vi "HW_Gantner_DAQ FGV.vi"(0 "DevName":string="Gantner", 1 "Oper.":T13, 2 "Path.ModuCFG":path, 5 "ActiveModuTag":string, 7 "TreePara":cluster{"ColHdrs":string[], "Items":string[][]}, 9 "DataBuf":refnum<queue>, 11 "error in":errorcluster caption="错误输入", 12 "ImportPara":T1(array[cluster])) -> (3 "Cfg out":T3[](array[typedef]), 4 "ActiveModuCHtype":string, 6 "Modu[] info":T2[](array[typedef]), 8 "ActiveCFG":T3, 10 "cfg change?":bool, 14 "TempCFG out":T3[](array[typedef]), 15 "error out":errorcluster caption="错误输出")   [LabVIEW 2016]
uses:
  DAQ FGV Operations.ctl
  Ctrls/HardWare _ Module Configuration.ctl
  Ctrls/HardWare _ Channel Parameters.ctl
  GantnerDriver/Gantner-Instruments HighSpeedPort/e.gate Configuration.ctl
  GantnerDriver/Gantner-Instruments HighSpeedPort/e.gate Channel Data.ctl
  GantnerDriver/Gantner-Instruments HighSpeedPort/e.gate Data Type.ctl
  GantnerDriver/Gantner-Instruments HighSpeedPort/e.gate Protocol Type.ctl
  GantnerDriver/Gantner-Instruments HighSpeedPort/e.gate Module  Data.ctl
  GantnerDriver/Gantner-Instruments HighSpeedPort/e.gateHSP_DLLhandle.ctl
  Gantner Device Info.ctl
  HW_Module Info.ctl
  Ctrls/HardWare Basic Info _ Channel.ctl
  X-DAQ Viewer/Controls/ConfigFGVCtrl.ctl
panel:
  in  "tempVari":T11={"DevName"="", "Usedcfg"=[], "TempCFG"=[], "ActiveModuIdx"=0, "SampRate"=0.0, "T0"=timestamp(0 s since 1904-01-01), "Path"={"ModuCFG_dflt"=path "", "ModuCFG_InUsed"=path ""}, "AllInUsedModu[]"=[], "Configuration"={"connection ID"=refnum, "IPAddress"="", "BufferIndex"=0, "StateMessage"="", "StateCode"=0, "HeaderSize"=0, "BufferSize"=0, "IsBigEndian"=0, "Version"=0, "ChannelCount"=0, "FrameLength"=0, "StartTime"=0.0, "dActTimeToSecondFactor"=0.0, "StartTimeToDayFactor"=0.0, "BufferFillRate"=0.0, "SampleRate"=0.0, "ChannelData"=[], "DecodeTimeFormat"="", "SummaryPath"="", "WithCheckSum"=0, "dActTimeDataType"=enum."NO", "MaxWriteCount"=0, "MaxReadCount"=0, "TempOffsetRead"=0, "TempLengthRead"=0, "Protocol"=enum."ASCII", "IsSupported"=0, "InputAccessList"=[], "OutputAccessList"=[], "DataSource"=enum."CircleBuffer", "Modules"=[], "DLL-Handle"={"clientInstance"=0, "connectionInstance"=0}}, "Iteration"=1000, "InUsedPhyCH[]"={"CHAlias"=[], "Unit"=[], "SampleRate"=[], "FilterFreq"=[], "SlopeA"=[], "InterceptB"=[], "SampMax"=[], "SampMin"=[], "AlarmMax"=[], "AlarmMin"=[], "Formula"=[]}, "StartT0"=timestamp(0 s since 1904-01-01), "Modu[] info"=[], "InUsedChanIdx[]"=[], "Wait (ms)"=500, "PhyChUsed[]"=[]} {"Configuration"."StartTime" format="%#.10f"; "Configuration"."dActTimeToSecondFactor" format="%#.10f"; "Configuration"."StartTimeToDayFactor" format="%#_10f"}
  in  "CFGinTree":T12
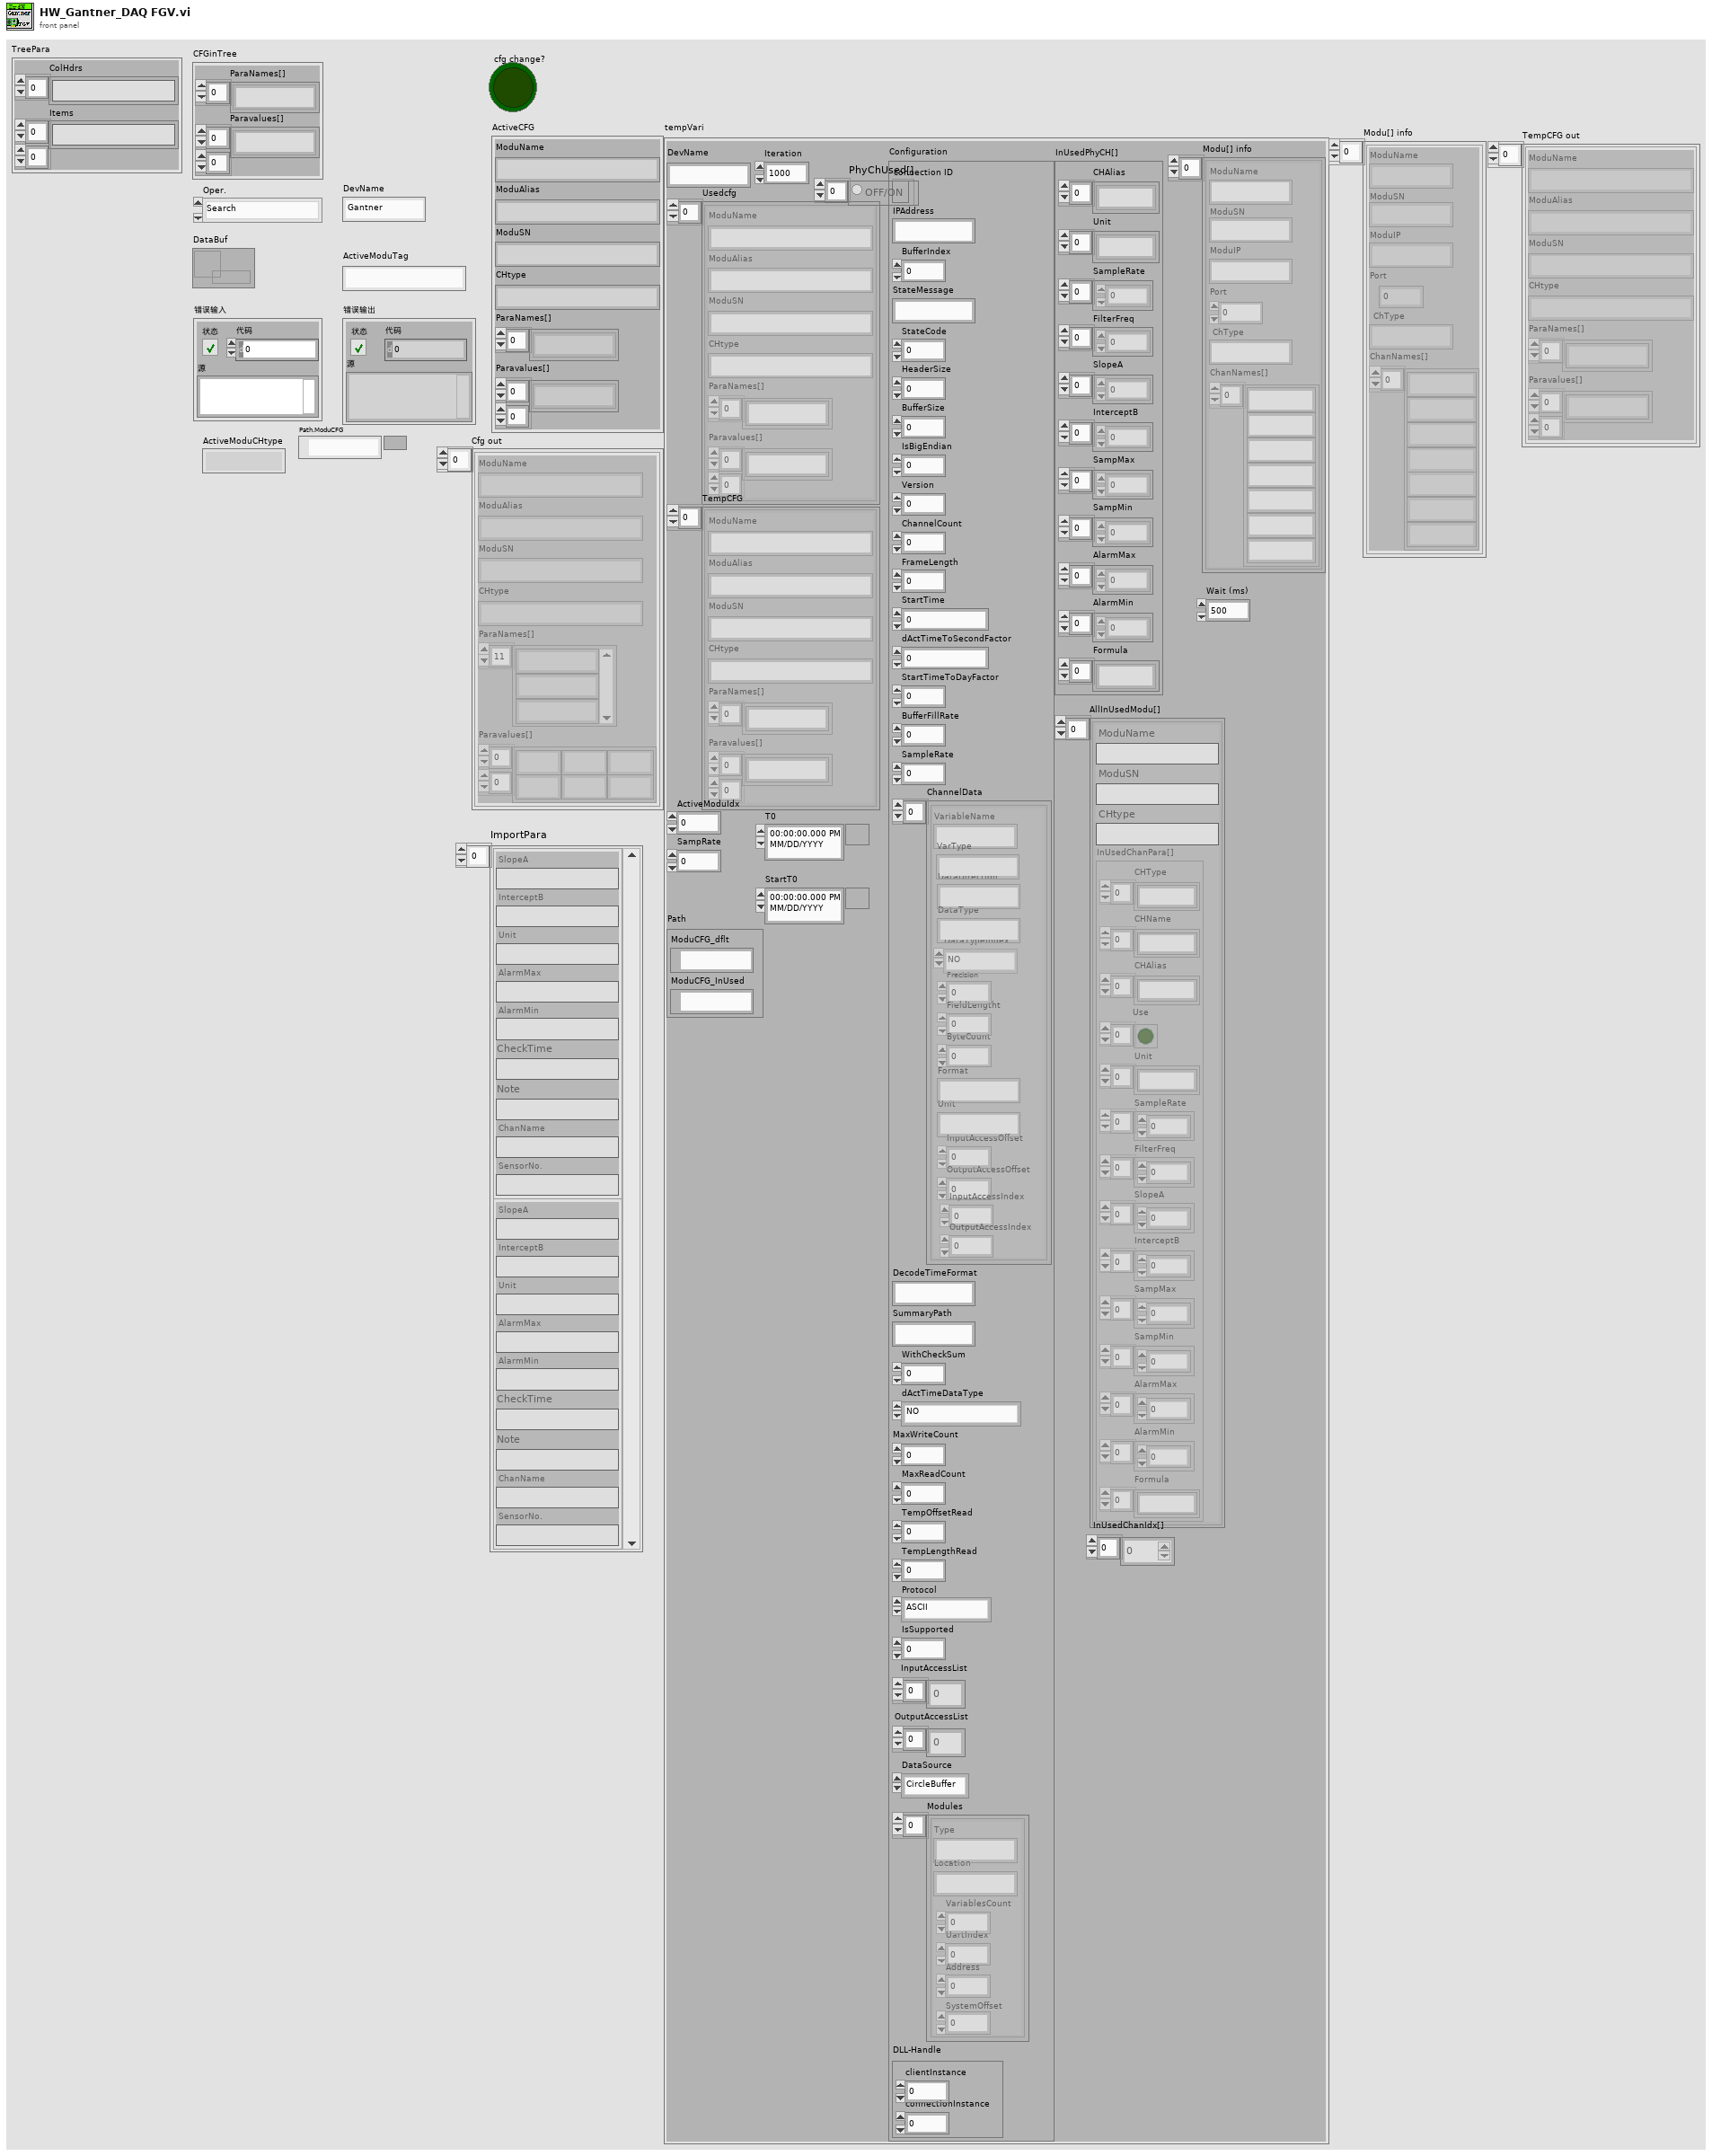
[diagram p1: front panel]
types:
  T1 = cluster{"SlopeA":string, "InterceptB":string, "Unit":string, "AlarmMax":string, "AlarmMin":string, "CheckTime":string, "Note":string, "ChanName":string, "SensorNo.":string}[]
  T2 = typedef "Gantner Device Info.ctl" = cluster{"ModuName":string, "ModuSN":string, "ModuIP":string, "Port":i32, "ChType":string, "ChanNames[]":string[]}
  T3 = typedef "HardWare _ Module Configuration.ctl" = cluster{"ModuName":string, "ModuAlias":string, "ModuSN":string, "CHtype":string, "ParaNames[]":string[], "Paravalues[]":string[][]}
  T4 = typedef "HardWare _ Channel Parameters.ctl" = cluster{"CHType":string[], "CHName":string[], "CHAlias":string[], "Use":bool[], "Unit":string[], "SampleRate":dbl[], "FilterFreq":dbl[], "SlopeA":dbl[], "InterceptB":dbl[], "SampMax":dbl[], "SampMin":dbl[], "AlarmMax":dbl[], "AlarmMin":dbl[], "Formula":string[]}
  T5 = typedef "e.gate Configuration.ctl" = cluster{"connection ID":refnum<k5>, "IPAddress":string, "BufferIndex":i32, "StateMessage":string, "StateCode":i8, "HeaderSize":i32, "BufferSize":i32, "IsBigEndian":i32, "Version":i32, "ChannelCount":i32, "FrameLength":i32, "StartTime":dbl, "dActTimeToSecondFactor":dbl, "StartTimeToDayFactor":dbl, "BufferFillRate":dbl, "SampleRate":dbl, "ChannelData":T6[], "DecodeTimeFormat":string, "SummaryPath":string, "WithCheckSum":i32, "dActTimeDataType":T7, "MaxWriteCount":i32, "MaxReadCount":i32, "TempOffsetRead":i32, "TempLengthRead":i32, "Protocol":T8, "IsSupported":i32, "InputAccessList":i32[], "OutputAccessList":i32[], "DataSource":enum16{"CircleBuffer", "test.con Logger", "test.con Archive"}, "Modules":T9[], "DLL-Handle":T10}
  T6 = typedef "e.gate Channel Data.ctl" = cluster{"VariableName":string, "DataDirection":string, "DataType":string, "DataTypeIndex":T7, "Precision":i16, "FieldLengtht":i16, "ByteCount":i32, "Format":string, "Unit":string, "InputAccessOffset":i32, "OutputAccessOffset":i16, "InputAccessIndex":i16, "OutputAccessIndex":i16, "VarType":string}
  T7 = typedef "e.gate Data Type.ctl" = enum16{"NO", "BOOL", "SINT8", "USINT8", "SINT16", "USINT16", "SINT32", "USINT32", "FLOAT", "SET8", "SET16", "SET32", "DOUBLE", "SINT64", "USINT64", "SET64"}
  T8 = typedef "e.gate Protocol Type.ctl" = enum16{"ASCII", "HighspeedPort Online", "HighspeedPort Buffer", "eGateHighspeedPortDLL "}
  T9 = typedef "e.gate Module  Data.ctl" = cluster{"Type":string, "Location":string, "VariablesCount":i16, "UartIndex":i16, "Address":i16, "SystemOffset":i16}
  T10 = typedef "e.gateHSP_DLLhandle.ctl" = cluster{"clientInstance":i32, "connectionInstance":i32}
  T11 = cluster{"DevName":string, "Usedcfg":T3[], "TempCFG":T3[], "ActiveModuIdx":i32, "SampRate":dbl, "T0":timestamp, "Path":cluster{"ModuCFG_dflt":path, "ModuCFG_InUsed":path}, "AllInUsedModu[]":cluster{"ModuName":string, "ModuSN":string, "CHtype":string, "InUsedChanPara[]":T4}[], "Configuration":T5, "Iteration":i32, "InUsedPhyCH[]":cluster{"CHAlias":string[], "Unit":string[], "SampleRate":dbl[], "FilterFreq":dbl[], "SlopeA":dbl[], "InterceptB":dbl[], "SampMax":dbl[], "SampMin":dbl[], "AlarmMax":dbl[], "AlarmMin":dbl[], "Formula":string[]}, "StartT0":timestamp, "Modu[] info":T2[], "InUsedChanIdx[]":i32[], "Wait (ms)":u32, "PhyChUsed[]":bool[]}
  T12 = cluster{"ParaNames[]":string[], "Paravalues[]":string[][]}
  T13 = typedef "DAQ FGV Operations.ctl" = enum16{"Search", "ReadCFG", "ReadVCH", "UpdateTempCFG", "DownloadCFG", "OpenCFG", "ImportPara", "Config", "Start", "Read", "Stop", "Clear"}
  T14 = typedef "ConfigFGVCtrl.ctl" = enum16{"Initialize", "Get Value", "Set Value", "Search Info"}
  T15 = typedef "HW_Module Info.ctl" = cluster{"ModName":string, "ModSN":string, "ChassisNo.":u32, "SlotNo.":u32, "ChanInfo":T16}
  T16 = typedef "HardWare Basic Info _ Channel.ctl" = cluster{"ChanType":string, "ChanNames[]":string[]}
  T17 = cluster{"DfltDataFolder":path, "ParaFolder":path, "SysCfg":path, "CHdef":path, "ModCfg":path, "DT Folder":path, "ErrorLog":path, "HBMlic":path, "HBMDriver":path}
  T18 = cluster{"SlopeA":string, "InterceptB":string, "Unit":string, "AlarmMax":string, "AlarmMin":string, "CheckTime":string, "Note":string, "ChanName":string, "SensorNo.":string}
  T19 = cluster{"ModuName":string, "ModuSN":string, "CHtype":string, "InUsedChanPara[]":T4}[]
  T20 = cluster{"ModuName":string, "ModuSN":string, "CHtype":string, "InUsedChanPara[]":T4}
  T21 = cluster{"CHAlias":string[], "Unit":string[], "SampleRate":dbl[], "FilterFreq":dbl[], "SlopeA":dbl[], "InterceptB":dbl[], "SampMax":dbl[], "SampMin":dbl[], "AlarmMax":dbl[], "AlarmMin":dbl[], "Formula":string[]}
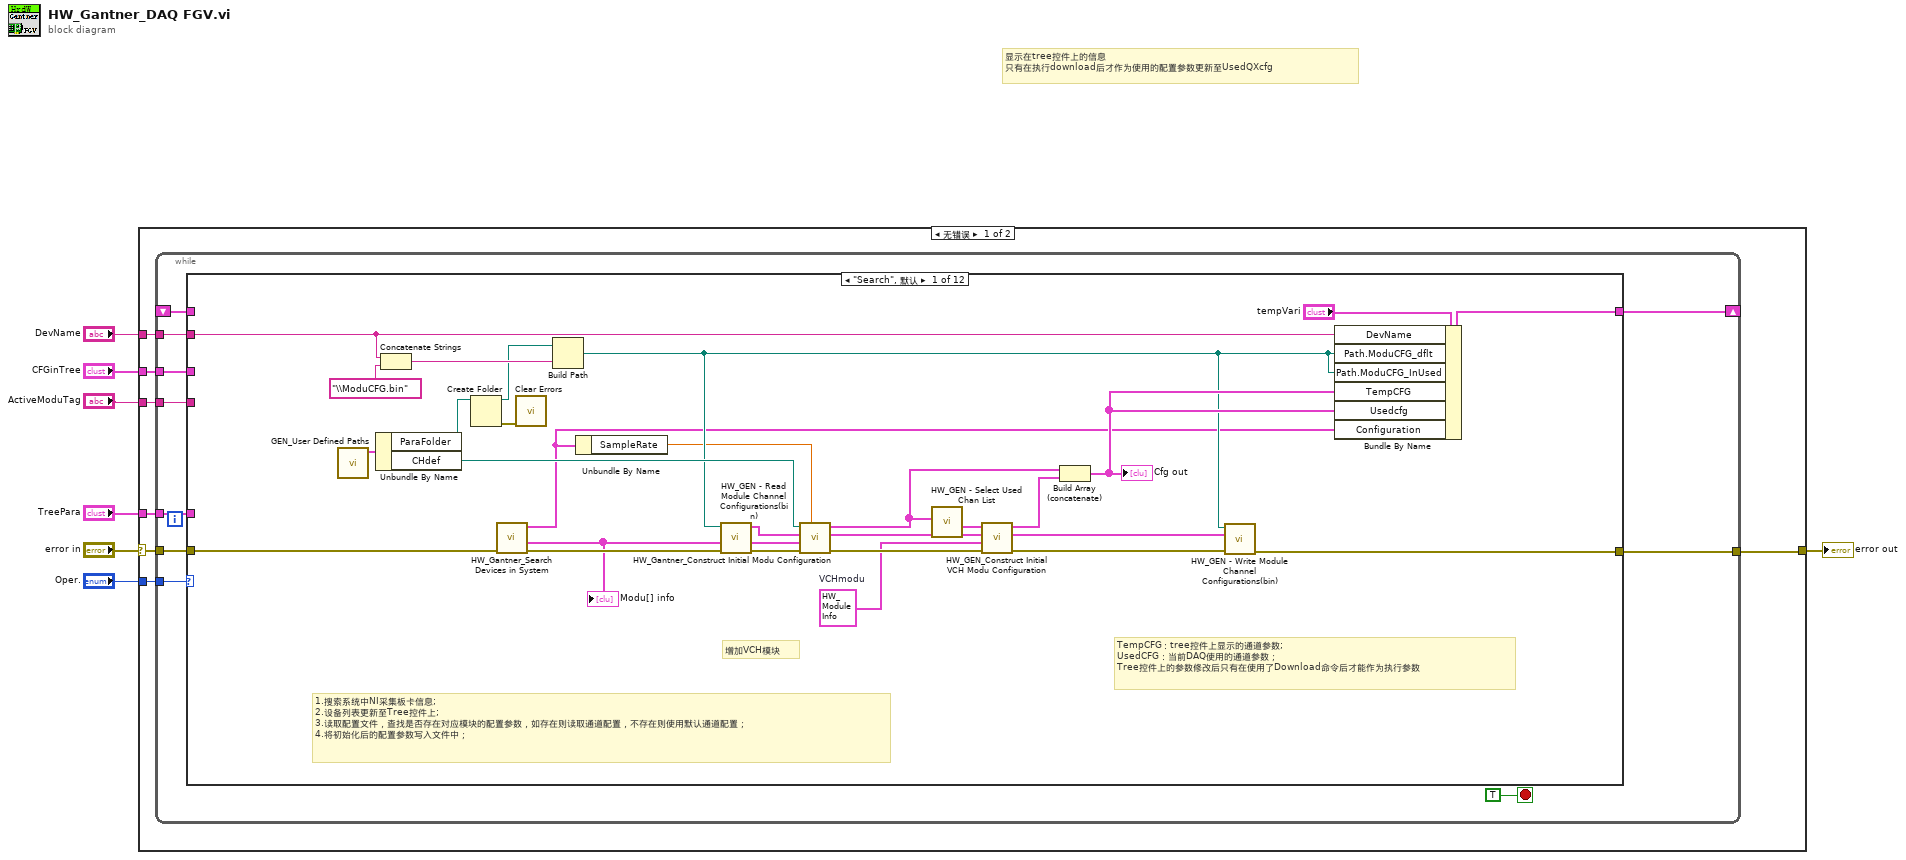
[diagram p0: block diagram]
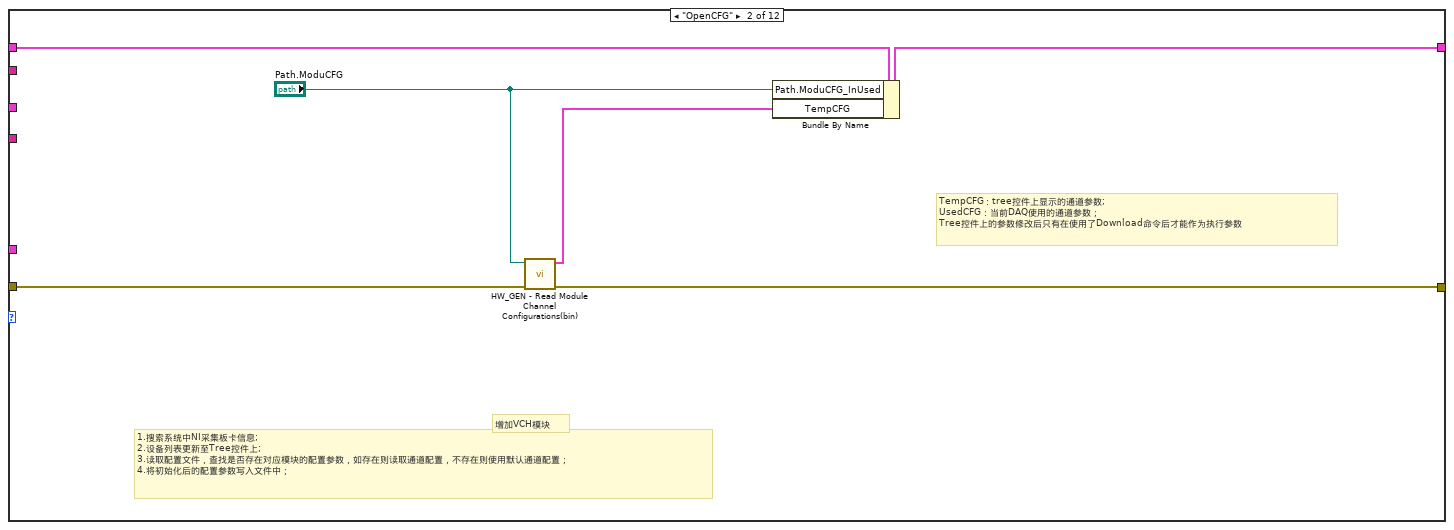
[diagram p2: hidden frame]
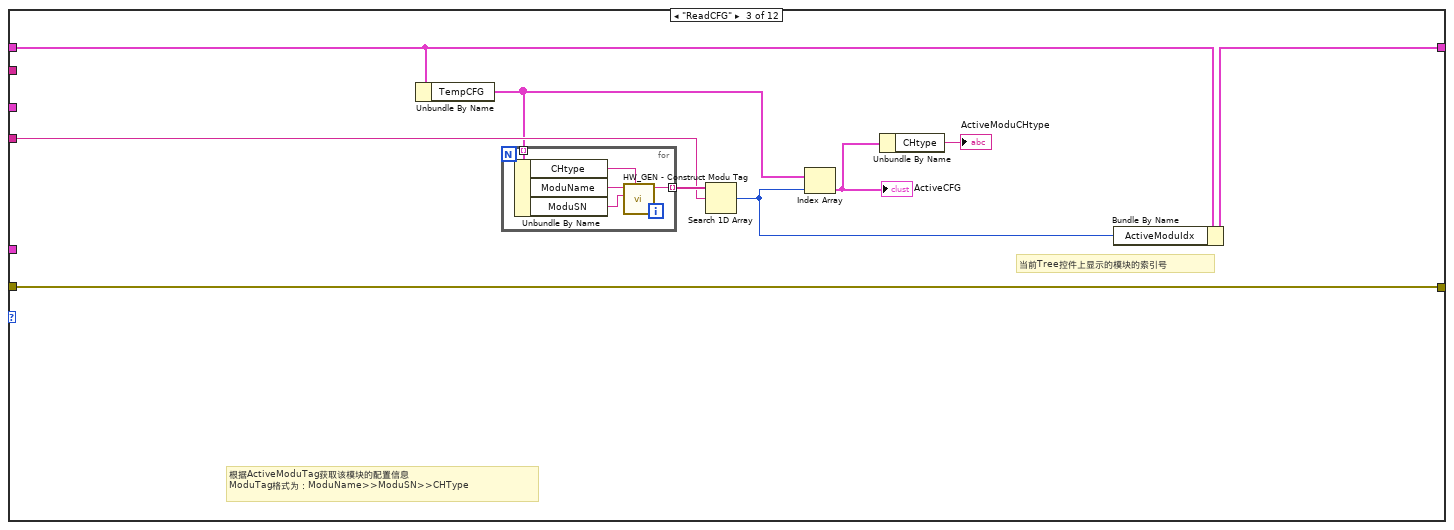
[diagram p3: hidden frame]
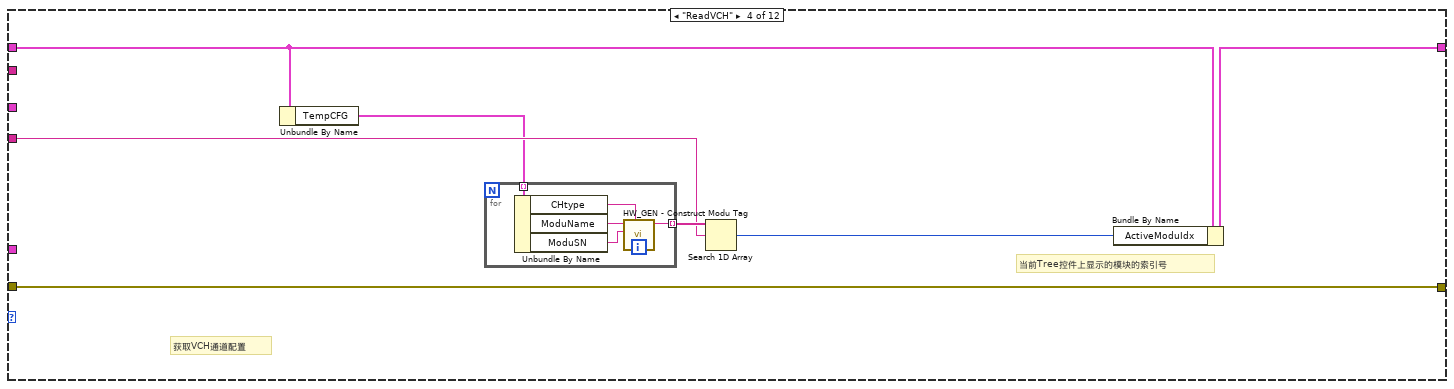
[diagram p4: hidden frame]
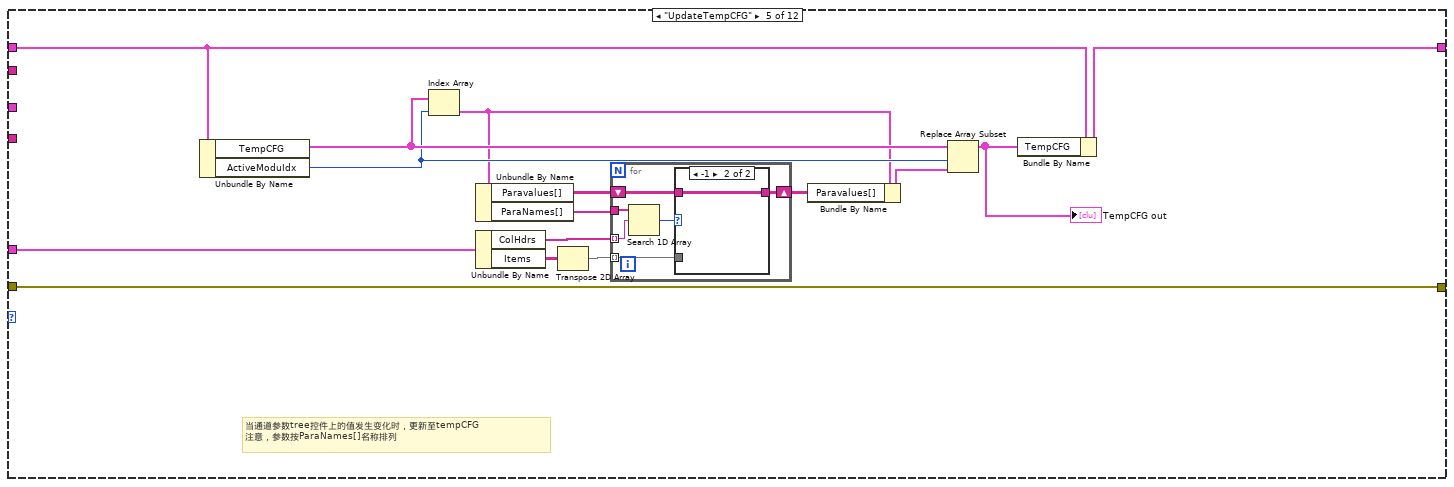
[diagram p5: hidden frame]
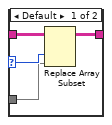
[diagram p6: hidden frame]
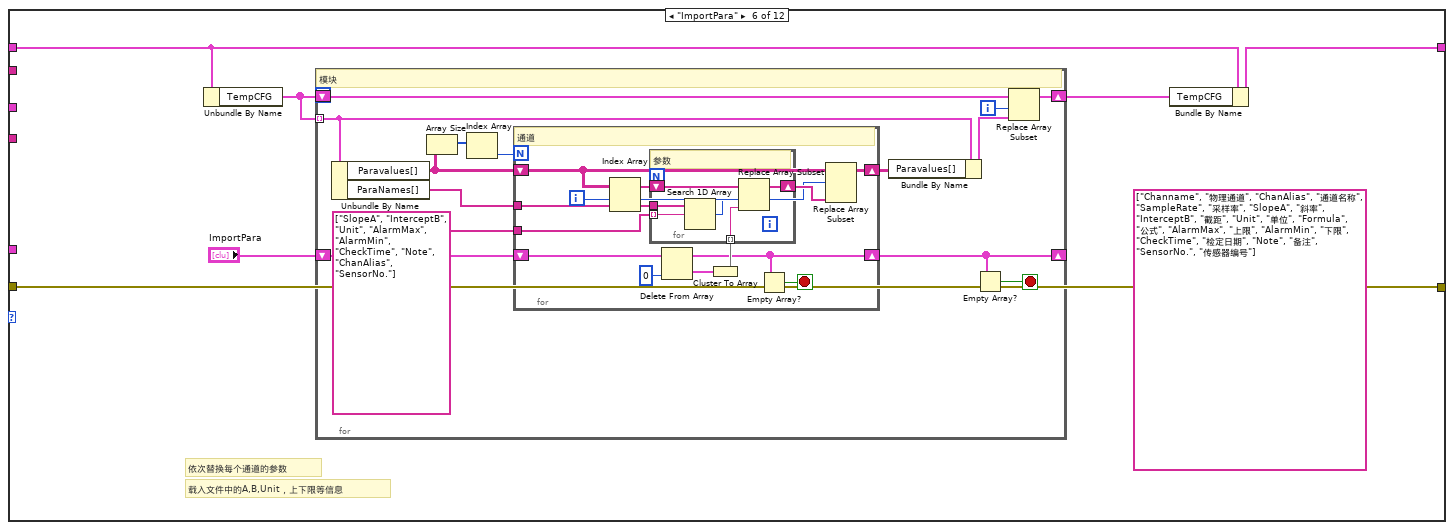
[diagram p7: hidden frame]
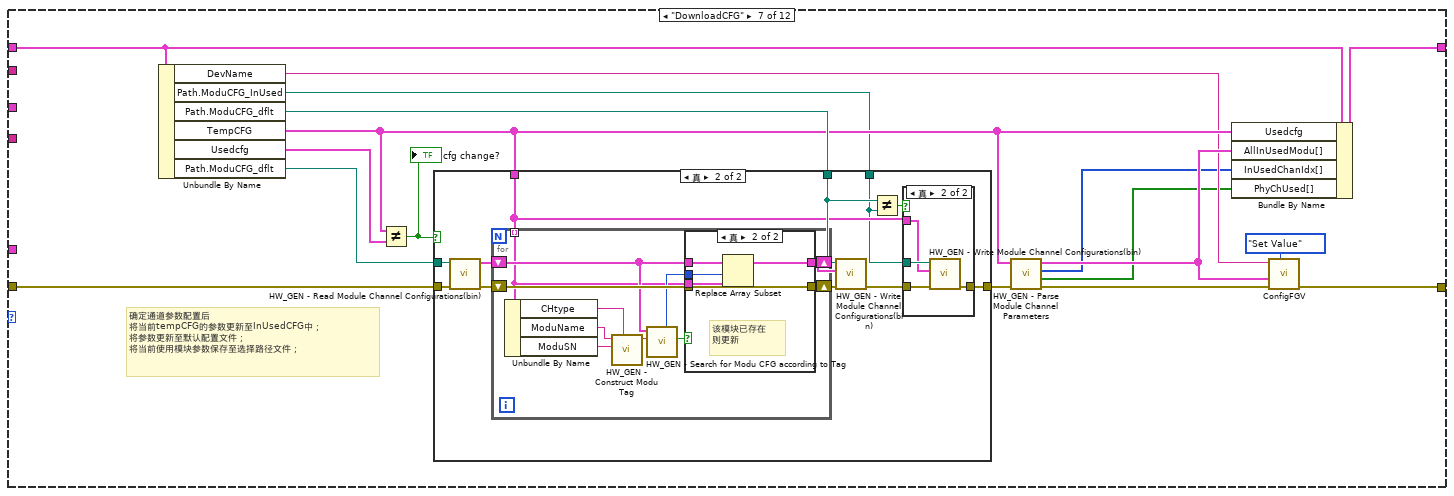
[diagram p8: hidden frame]
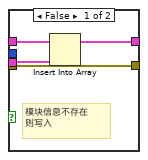
[diagram p11: hidden frame]
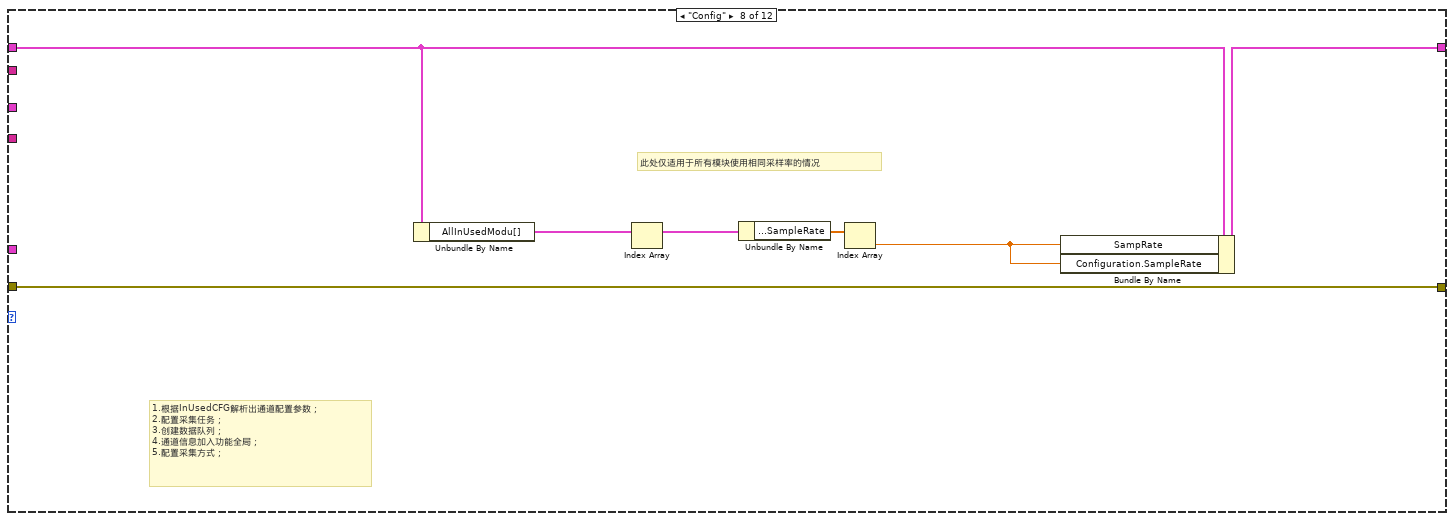
[diagram p12: hidden frame]
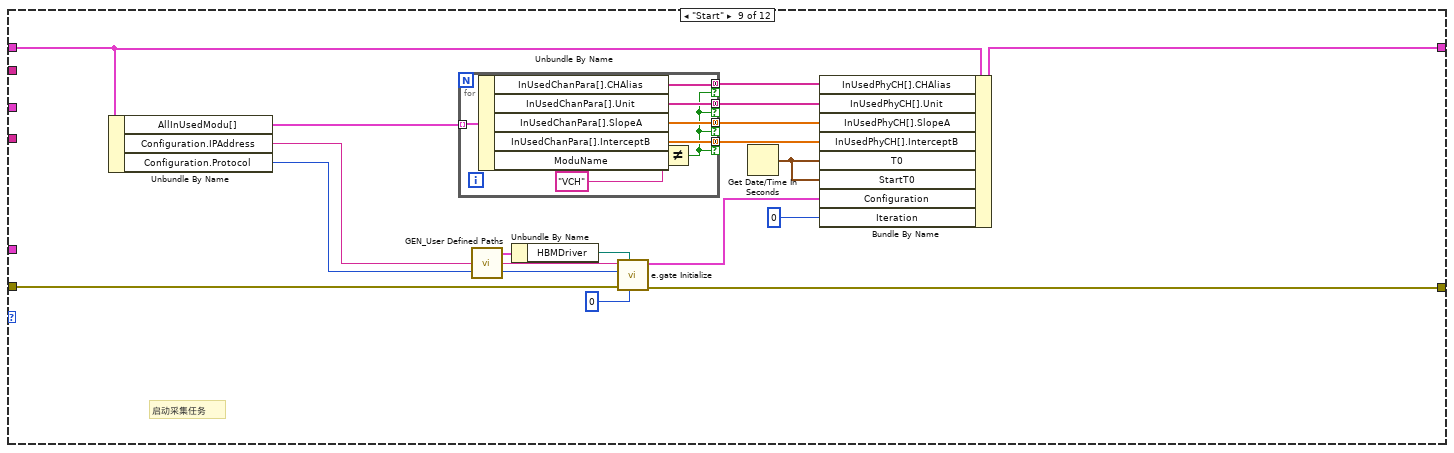
[diagram p13: hidden frame]
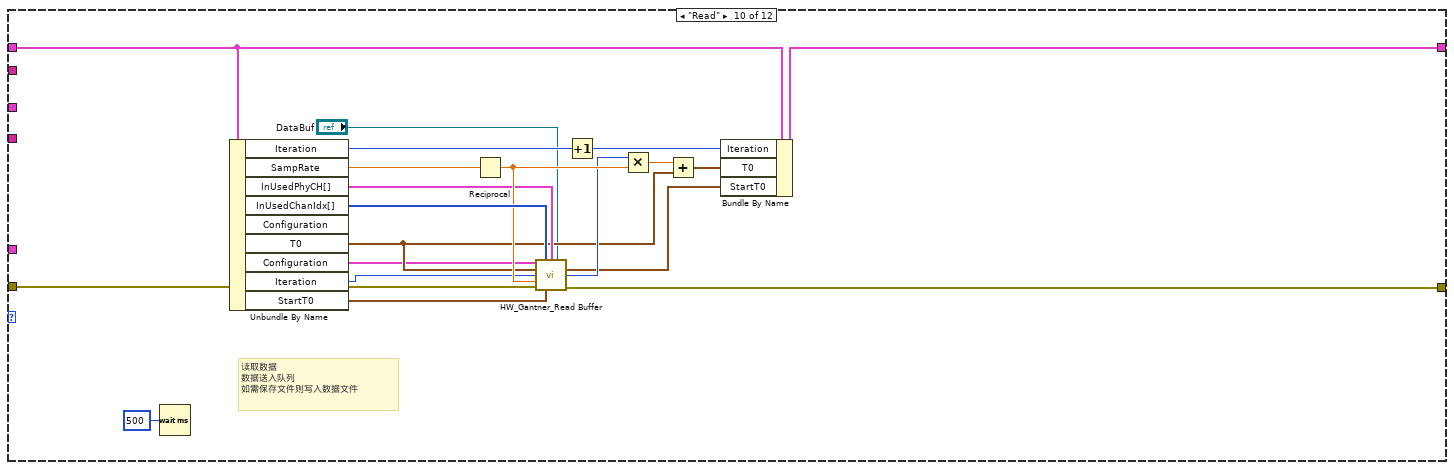
[diagram p14: hidden frame]
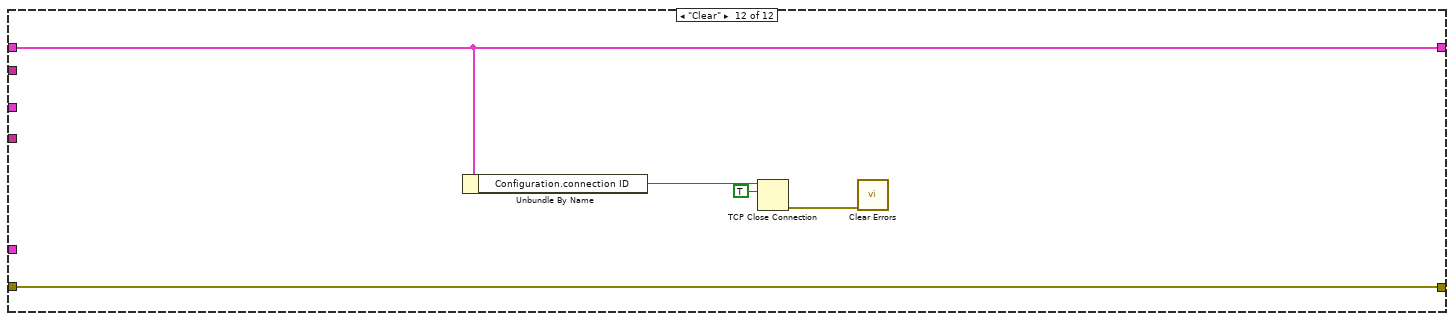
[diagram p16: hidden frame]
diagram:
  # "显示在tree控件上的信息\n只有在执行download后才作为使用的配置参数更新至UsedQXcfg"
  n1 = case shown="无错误" "error in" {
    selector: "error in" -> [w13 w263]
    tunnel: [w9 w263] -> w6
    tunnel: "Oper." -> [w14 _]
    tunnel: "ActiveModuTag" -> [w12 _]
    tunnel: "CFGinTree" -> [w11 _]
    tunnel: "TreePara" -> [w10 _]
    tunnel: "DevName" -> [w8 _]
    frame No Error {
      n2 = while {
        tunnel: w14 -> [w23]
        tunnel: w13 -> [w22]
        tunnel: w12 -> [w21]
        tunnel: w11 -> [w20]
        tunnel: w10 -> [w19]
        tunnel: [w18] -> w9
        shift-right: [w17] -> _
        shift-left: _ -> [w16]
        tunnel: w8 -> [w15]
        stop <- TRUE stop-if-true
        n3 = case shown="\"Search\", 默认" w23 {
          tunnel: w22 -> [w44 w57 w67 w79 w99 w116 w163 w210 w220 w249 w257 w262]
          tunnel: w21 -> [_ _ w65 w77 _ _ _ _ _ _ _ _]
          tunnel: w20 -> [_ _ _ _ _ _ _ _ _ _ _ _]
          tunnel: w19 -> [_ _ _ _ w97 _ _ _ _ _ _ _]
          tunnel: [w50 w54 w67 w79 w99 w116 w155 w210 w219 w250 w257 w262] -> w18
          tunnel: [w48 w58 w61 w73 w93 w114 w165 w209 w227 w254 w256 w261] -> w17
          tunnel: w16 -> [_ w55 w62 w74 w98 w115 w166 w208 w226 w255 w256 w261]
          tunnel: w15 -> [w45 _ _ _ _ _ _ _ _ _ _ _]
          frame "Search", Default {
            w25 = T15 {"ModName"="VCH", "ModSN"="VCH", "ChassisNo."=0, "SlotNo."=0, "ChanInfo"={"ChanType"="VCH", "ChanNames[]"=["VCH0", "VCH1", "VCH2", "VCH3", "VCH4", "VCH5", "VCH6", "VCH7"]}}  # VCHmodu
            # "增加VCH模块"
            # "TempCFG：tree控件上显示的通道参数;\nUsedCFG：当前DAQ使用的通道参数；\nTree控件上的参数修改后只有在使用了Download命令后才能作为执行参数"
            # "1.搜索系统中NI采集板卡信息;\n2.设备列表更新至Tree控件上;\n3.读取配置文件，查找是否存在对应模块的配置参数，如存在则读取通道配置，不存在则使用默认通道配置；\n4.将初始化后的配置参数写入文件中；"
            n4 = call "GEN_User Defined Paths.vi"() -> ("UserDefinedPath"=w52:T17)  [unwired: 11 in]
            n5 = Unbundle By Name(w52) -> ("ParaFolder"=w32:path, "CHdef"=w42:path)
            n6 = Concatenate Strings(w45, "\\ModuCFG.bin") -> (w31:string)
            n7 = Create Folder(path (use dialog)=w32) -> (created path=w30:path, error out=w33:errorcluster)  [unwired: 2 in, 1 out]
            n8 = call "HW_Gantner_Search Devices in System.vi"("error in"=w44) -> ("error out"=w46:errorcluster, "Modu[] info"=w26:T2[], "Configuration out"=w28:T5)  [unwired: 8 in]
            "Modu[] info" <- w26
            n9 = call <vilib>:"Clear Errors.vi"("error in (no error)"=w33) -> ()  [unwired: 5 in, 2 out]
            n10 = Build Path(base path=w30, name or relative path=w31) -> (appended path=w29:path)
            n11 = Unbundle By Name(w28) -> ("SampleRate"=w27:dbl)
            n12 = call "HW_GEN - Read Module Channel Configurations(bin).vi"("error in"=w46, "ModuCFG path"=w29) -> ("error out"=w51:errorcluster, "ModCFG out"=w41:T3[])  [unwired: 8 in]
            n13 = call "HW_Gantner_Construct Initial Modu Configuration.vi"("SampleRate"=w27, "error in"=w51, "Modu[] in"=w26, "ModCFG in"=w41, "CHdef"=w42) -> ("error out"=w43:errorcluster, "ModCFG to File"=w40:T3[], "ModuInSysCFG"=w35:T3[])  [unwired: 4 in]
            n14 = call "HW_GEN - Select Used Chan List.vi"("Cfg in"=w35) -> ("VarList"=w34:cluster{"Tag":string[], "Alias":string[]})  [unwired: 9 in, 1 out]
            n15 = call "HW_GEN_Construct Initial VCH Modu Configuration.vi"("error in"=w43, "VCHmodu"=w25, "ModCFG in"=w40, "VarList"=w34) -> ("error out"=w38:errorcluster, "ModCFG to File"=w39:T3[], "ModuCFG out"=w37:T3)  [unwired: 5 in]
            n16 = Build Array (concatenate)(w35, w37) -> (w36:T3[])
            "Cfg out" <- w36
            n17 = call "HW_GEN - Write Module Channel Configurations(bin).vi"("error in"=w38, "ModuCfg"=w39, "Path"=w29) -> ("error out"=w50:errorcluster)  [unwired: 8 in]
            n18 = Bundle By Name(cluster="tempVari", "DevName"=w45, "Path.ModuCFG_dflt"=w29, "Path.ModuCFG_InUsed"=w29, "TempCFG"=w36, "Usedcfg"=w36, "Configuration"=w28) -> (w48:T11)
          }
          frame "OpenCFG" {
            # "增加VCH模块"
            # "TempCFG：tree控件上显示的通道参数;\nUsedCFG：当前DAQ使用的通道参数；\nTree控件上的参数修改后只有在使用了Download命令后才能作为执行参数"
            # "1.搜索系统中NI采集板卡信息;\n2.设备列表更新至Tree控件上;\n3.读取配置文件，查找是否存在对应模块的配置参数，如存在则读取通道配置，不存在则使用默认通道配置；\n4.将初始化后的配置参数写入文件中；"
            n19 = call "HW_GEN - Read Module Channel Configurations(bin).vi"("error in"=w57, "ModuCFG path"="Path.ModuCFG") -> ("error out"=w54:errorcluster, "ModCFG out"=w53:T3[])  [unwired: 8 in]
            n20 = Bundle By Name(cluster=w55, "Path.ModuCFG_InUsed"="Path.ModuCFG", "TempCFG"=w53) -> (w58:T11)
          }
          frame "ReadCFG" {
            # "当前Tree控件上显示的模块的索引号"
            # "根据ActiveModuTag获取该模块的配置信息\nModuTag格式为：ModuName>>ModuSN>>CHType"
            n21 = Unbundle By Name(w62) -> ("TempCFG"=w64:T3[])
            n22 = for {
              tunnel: w64 -> [w72] mode=indexing
              tunnel: [w68] -> w66 mode=indexing
              n23 = Unbundle By Name(w72) -> ("CHtype"=w71:string, "ModuName"=w70:string, "ModuSN"=w69:string)
              n24 = call "HW_GEN - Construct Modu Tag.vi"("ChanType"=w71, "ModSN"=w69, "ModName"=w70) -> ("String"=w68:string)  [unwired: 8 in]
            }
            n25 = Search 1D Array(1D array=w66, element=w65) -> (index of element=w63:i32)  [unwired: 1 in]
            n26 = Index Array(array=w64, index=w63) -> (element=w60:T3)
            "ActiveCFG" <- w60
            n27 = Unbundle By Name(w60) -> ("CHtype"=→"ActiveModuCHtype":string)
            n28 = Bundle By Name(cluster=w62, "ActiveModuIdx"=w63) -> (w61:T11)
          }
          frame "ReadVCH" {
            # "当前Tree控件上显示的模块的索引号"
            # "获取VCH通道配置"
            n29 = Unbundle By Name(w74) -> ("TempCFG"=w76:T3[])
            n30 = for {
              tunnel: w76 -> [w84] mode=indexing
              tunnel: [w80] -> w78 mode=indexing
              n31 = Unbundle By Name(w84) -> ("CHtype"=w83:string, "ModuName"=w82:string, "ModuSN"=w81:string)
              n32 = call "HW_GEN - Construct Modu Tag.vi"("ChanType"=w83, "ModSN"=w81, "ModName"=w82) -> ("String"=w80:string)  [unwired: 8 in]
            }
            n33 = Search 1D Array(1D array=w78, element=w77) -> (index of element=w75:i32)  [unwired: 1 in]
            n34 = Bundle By Name(cluster=w74, "ActiveModuIdx"=w75) -> (w73:T11)
          }
          frame "UpdateTempCFG" {
            # "当通道参数tree控件上的值发生变化时，更新至tempCFG\n注意，参数按ParaNames[]名称排列"
            n35 = Unbundle By Name(w98) -> ("TempCFG"=w96:T3[], "ActiveModuIdx"=w95:i32)
            n36 = Index Array(array=w96, index=w95) -> (element=w92:T3)
            n37 = Unbundle By Name(w92) -> ("Paravalues[]"=w88:string[][], "ParaNames[]"=w91:string[])
            n38 = Unbundle By Name(w97) -> ("ColHdrs"=w90:string[], "Items"=w89:string[][])
            n39 = Transpose 2D Array(2D array=w89) -> (transposed array=w87:string[][])
            n40 = for {
              tunnel: w91 -> [w104]
              tunnel: w90 -> [w103] mode=indexing
              tunnel: w87 -> [w105] mode=indexing
              shift-right: [w100] -> w86
              shift-left: w88 -> [w101]
              n41 = Search 1D Array(1D array=w104, element=w103) -> (index of element=w102:i32)  [unwired: 1 in]
              n42 = case shown="-1" w102 {
                selector: w102 -> [w107 _]
                tunnel: w105 -> [w106 _]
                tunnel: w101 -> [w109 w110]
                tunnel: [w108 w110] -> w100
                frame Default {
                  n43 = Replace Array Subset(array=w109, new element=w106, index (col)=w107) -> (w108:string[][])  [unwired: 1 in]
                }
                frame -1 {
                }
              }
            }
            n44 = Bundle By Name(cluster=w92, "Paravalues[]"=w86) -> (w94:T3)
            n45 = Replace Array Subset(array=w96, new element=w94, index=w95) -> (w85:T3[])
            "TempCFG out" <- w85
            n46 = Bundle By Name(cluster=w98, "TempCFG"=w85) -> (w93:T11)
          }
          frame "ImportPara" {
            (unwired) string[][] [["Channame", "物理通道"], ["ChanAlias", "通道名称"], ["SampleRate", "采样率"], ["SlopeA", "斜率"], ["InterceptB", "截距"], ["Unit", "单位"], ["Formula", "公式"], ["AlarmMax", "上限"], ["AlarmMin", "下限"], ["CheckTime", "检定日期"], ["Note", "备注"], ["SensorNo.", "传感器编号"]] ("DisCols[]")
            # "依次替换每个通道的参数"
            # "载入文件中的A,B,Unit，上下限等信息"
            n47 = Unbundle By Name(w115) -> ("TempCFG"=w111:T3[])
            n48 = for {
              shift-right: [w127] -> w113
              shift-left: w111 -> [w130]
              shift-right: [w121] -> _
              shift-left: "ImportPara" -> [w126]
              tunnel: w111 -> [w122] mode=indexing
              i -> [w129]
              stop <- w120 stop-if-true
              # "模块"
              n49 = Unbundle By Name(w122) -> ("Paravalues[]"=w119:string[][], "ParaNames[]"=w125:string[])
              n50 = Array Size(array=w119) -> (size(s)=w118:i32[])
              n51 = Index Array(array=w118) -> (element=w117:i32)  [unwired: 1 in]
              n52 = for {
                N: w117 -> [_]
                tunnel: w125 -> [w142]
                tunnel: string[] ["SlopeA", "InterceptB", "Unit", "AlarmMax", "AlarmMin", "CheckTime", "Note", "ChanAlias", "SensorNo."] ("ParaNames[]") -> [w141]
                shift-right: [w137] -> w121
                shift-left: w126 -> [w143]
                shift-right: [w132] -> w123
                shift-left: w119 -> [w134]
                i -> [w131]
                stop <- w136 stop-if-true
                # "通道"
                n53 = Index Array(array=w134, index (row)=w131) -> (element=w135:string[])  [unwired: 1 in]
                n54 = Delete From Array(array=w143, index=0) -> (deleted portion=w139:T18, array with subset deleted=w137:T1)  [unwired: 1 in]
                n55 = Cluster To Array(cluster=w139) -> (array=w140:string[])
                n56 = for {
                  tunnel: w142 -> [w149]
                  tunnel: w141 -> [w148] mode=indexing
                  tunnel: w140 -> [w146] mode=indexing
                  shift-right: [w145] -> w133
                  shift-left: w135 -> [w147]
                  # "参数"
                  n57 = Search 1D Array(1D array=w149, element=w148) -> (index of element=w144:i32)  [unwired: 1 in]
                  n58 = Replace Array Subset(array=w147, new element=w146, index=w144) -> (w145:string[])
                }
                n59 = Empty Array?(array=w137) -> (empty?=w136:bool)
                n60 = Replace Array Subset(array=w134, new element=w133, index (row)=w131) -> (w132:string[][])  [unwired: 1 in]
              }
              n61 = Bundle By Name(cluster=w122, "Paravalues[]"=w123) -> (w128:T3)
              n62 = Empty Array?(array=w121) -> (empty?=w120:bool)
              n63 = Replace Array Subset(array=w130, new element=w128, index=w129) -> (w127:T3[])
            }
            n64 = Bundle By Name(cluster=w115, "TempCFG"=w113) -> (w114:T11)
          }
          frame "DownloadCFG" {
            # "确定通道参数配置后\n将当前tempCFG的参数更新至InUsedCFG中；\n将参数更新至默认配置文件；\n将当前使用模块参数保存至选择路径文件；"
            n65 = Unbundle By Name(w166) -> ("DevName"=w153:string, "Path.ModuCFG_InUsed"=w152:path, "Path.ModuCFG_dflt"=w160:path, "TempCFG"=w158:T3[], "Usedcfg"=w164:T3[], "Path.ModuCFG_dflt"=w162:path)
            n66 = Not Equal?(x=w158, y=w164) -> (x != y?=w161:bool)
            "cfg change?" <- w161
            n67 = case shown="真" w161 {
              tunnel: w163 -> [_ w178]
              tunnel: w162 -> [_ w177]
              tunnel: w158 -> [_ w169]
              tunnel: w160 -> [_ w170]
              tunnel: w152 -> [_ w168]
              tunnel: [_ w167] -> w159
              frame False {
              }
              frame True {
                n68 = call "HW_GEN - Read Module Channel Configurations(bin).vi"("error in"=w178, "ModuCFG path"=w177) -> ("error out"=w175:errorcluster, "ModCFG out"=w176:T3[])  [unwired: 8 in]
                n69 = for {
                  shift-right: [w188] -> w174
                  shift-left: w175 -> [w193]
                  tunnel: w169 -> [w190] mode=indexing
                  shift-right: [w189] -> w173
                  shift-left: w176 -> [w191]
                  n70 = Unbundle By Name(w190) -> ("CHtype"=w187:string, "ModuName"=w186:string, "ModuSN"=w185:string)
                  n71 = call "HW_GEN - Construct Modu Tag.vi"("ChanType"=w187, "ModSN"=w185, "ModName"=w186) -> ("String"=w184:string)  [unwired: 8 in]
                  n72 = call "HW_GEN - Search for Modu CFG according to Tag.vi"("ModuTag"=w184, "ModuCFG[]"=w191) -> ("find?"=w194:bool, "idx"=w192:i32)  [unwired: 7 in, 1 out]
                  n73 = case shown="真" w194 {
                    tunnel: w193 -> [w197 w199]
                    tunnel: w192 -> [_ w202]
                    tunnel: w191 -> [w198 w203]
                    tunnel: w190 -> [w195 w201]
                    tunnel: [w196 w200] -> w189
                    tunnel: [w197 w199] -> w188
                    frame False {
                      # "模块信息不存在\n则写入"
                      n74 = Insert Into Array(array=w198, new element=w195) -> (w196:T3[])  [unwired: 1 in]
                    }
                    frame True {
                      # "该模块已存在\n则更新"
                      n75 = Replace Array Subset(array=w203, new element=w201, index=w202) -> (w200:T3[])
                    }
                  }
                }
                n76 = call "HW_GEN - Write Module Channel Configurations(bin).vi"("error in"=w174, "ModuCfg"=w173, "Path"=w170) -> ("error out"=w172:errorcluster)  [unwired: 8 in]
                n77 = Not Equal?(x=w170, y=w168) -> (x != y?=w171:bool)
                n78 = case shown="真" w171 {
                  tunnel: w172 -> [w179 w183]
                  tunnel: w169 -> [_ w181]
                  tunnel: w168 -> [_ w182]
                  tunnel: [w179 w180] -> w167
                  frame False {
                  }
                  frame True {
                    n79 = call "HW_GEN - Write Module Channel Configurations(bin).vi"("error in"=w183, "ModuCfg"=w181, "Path"=w182) -> ("error out"=w180:errorcluster)  [unwired: 8 in]
                  }
                }
              }
            }
            n80 = call "HW_GEN - Parse Module Channel Parameters.vi"("error in"=w159, "Usedcfg"=w158) -> ("error out"=w156:errorcluster, "PhyChUsed[]"=w150:bool[], "InUsedChanIdx[]"=w151:i32[], "AllInUsedModu[]"=w154:T19)  [unwired: 6 in]
            n81 = Bundle By Name(cluster=w166, "Usedcfg"=w158, "AllInUsedModu[]"=w154, "InUsedChanIdx[]"=w151, "PhyChUsed[]"=w150) -> (w165:T11)
            n82 = call "ConfigFGV.vi"("Command"=ConfigFGVCtrl."Set Value", "error in"=w156, "AllInUsedModu[]"=w154, "DevName"=w153) -> ("error out"=w155:errorcluster)  [unwired: 3 in, 4 out]
          }
          frame "Config" {
            # "此处仅适用于所有模块使用相同采样率的情况"
            # "1.根据InUsedCFG解析出通道配置参数；\n2.配置采集任务；\n3.创建数据队列；\n4.通道信息加入功能全局；\n5.配置采集方式；"
            n83 = Unbundle By Name(w208) -> ("AllInUsedModu[]"=w205:T19)
            n84 = Index Array(array=w205) -> (element=w207:T20)  [unwired: 1 in]
            n85 = Unbundle By Name(w207) -> ("InUsedChanPara[].SampleRate"=w206:dbl[])
            n86 = Index Array(array=w206) -> (element=w204:dbl)  [unwired: 1 in]
            n87 = Bundle By Name(cluster=w208, "SampRate"=w204, "Configuration.SampleRate"=w204) -> (w209:T11)
          }
          frame "Start" {
            # "启动采集任务"
            n88 = Unbundle By Name(w226) -> ("AllInUsedModu[]"=w225:T19, "Configuration.IPAddress"=w218:string, "Configuration.Protocol"=w217:T8)
            n89 = for {
              tunnel: w225 -> [w235] mode=indexing
              tunnel: [w233] -> w223 mode=concatenating if=w228
              tunnel: [w231] -> w224 mode=concatenating if=w228
              tunnel: [w230] -> w221 mode=concatenating if=w228
              tunnel: [w229] -> w222 mode=concatenating if=w228
              n90 = Unbundle By Name(w235) -> ("InUsedChanPara[].CHAlias"=w230:string[], "InUsedChanPara[].Unit"=w229:string[], "InUsedChanPara[].SlopeA"=w233:dbl[], "InUsedChanPara[].InterceptB"=w231:dbl[], "ModuName"=w232:string)
              n91 = Not Equal?(x=w232, y="VCH" ("x")) -> (x != y?=w228:bool)
            }
            n92 = call "GEN_User Defined Paths.vi"() -> ("UserDefinedPath"=w214:T17)  [unwired: 11 in]
            n93 = Unbundle By Name(w214) -> ("HBMDriver"=w213:path)
            n94 = call "e.gate Initialize.vi"("Buffer Index"=0, "eGateHighspeedPortDLLDLL Path"=w213, "error in (no error)"=w220, "Protocol"=w217, "IP Address"=w218) -> ("error out"=w219:errorcluster, "e.gate Configuration"=w212:T5)  [unwired: 5 in]
            n95 = Get Date/Time In Seconds() -> (seconds since 1Jan1904=w216:timestamp)
            n96 = Bundle By Name(cluster=w226, "InUsedPhyCH[].CHAlias"=w221, "InUsedPhyCH[].Unit"=w222, "InUsedPhyCH[].SlopeA"=w223, "InUsedPhyCH[].InterceptB"=w224, "T0"=w216, "StartT0"=w216, "Configuration"=w212, "Iteration"=0) -> (w227:T11)
          }
          frame "Read" {
            # "读取数据\n数据送入队列\n如需保存文件则写入数据文件"
            n97 = Wait (ms)(milliseconds to wait=u32 500) -> ()  [unwired: 1 out]
            n98 = Unbundle By Name(w255) -> ("Iteration"=w241:i32, "SampRate"=w239:dbl, "InUsedPhyCH[]"=w245:T21, "InUsedChanIdx[]"=w247:i32[], "T0"=w243:timestamp, "Configuration"=w237:T5, "Iteration"=w242:i32, "StartT0"=w240:timestamp)  [unwired: 1 out]
            n99 = Reciprocal(x=w239) -> (1/x=w246:dbl)
            n100 = call "HW_Gantner_Read Buffer.vi"("e.gate Configuration In"=w237, "InUsedChanIdx[]"=w247, "InUsedPhyCH[]"=w245, "DataBuf"="DataBuf", "CurrentT0"=w243, "Iteration"=w242, "dt"=w246, "error in"=w249, "StartT0"=w240) -> ("StartT0 out"=w238:timestamp, "data length"=w244:i32, "error out"=w250:errorcluster)  [unwired: 3 in, 1 out]
            n101 = Increment(x=w241) -> (x+1=w253:i32)
            n102 = Multiply(x=w244, y=w246) -> (x*y=w252:dbl)
            n103 = Add(x=w252, y=w243) -> (x+y=w251:timestamp)
            n104 = Bundle By Name(cluster=w255, "Iteration"=w253, "T0"=w251, "StartT0"=w238) -> (w254:T11)
          }
          frame "Stop" {
          }
          frame "Clear" {
            n105 = Unbundle By Name(w261) -> ("Configuration.connection ID"=w259:refnum<k5>)
            n106 = TCP Close Connection(connection ID=w259, abort (F)=TRUE ("中止(F)")) -> (error out=w258:errorcluster)  [unwired: 1 in, 1 out]
            n107 = call <vilib>:"Clear Errors.vi"("error in (no error)"=w258) -> ()  [unwired: 5 in, 2 out]
          }
        }
      }
    }
    frame Error {
    }
  }
  "error out" <- w6
